vi "set_PulseWidth_subvi.vi"(8 "error in (no error)":errorcluster, 9 "Pulsewidth":dbl, 10 "Aardvark Handle":i32 min=0, 11 "Address (0x50) in":u16=80 max=1023 format="%.0x") -> (0 "error out":errorcluster)   [LabVIEW 2014]
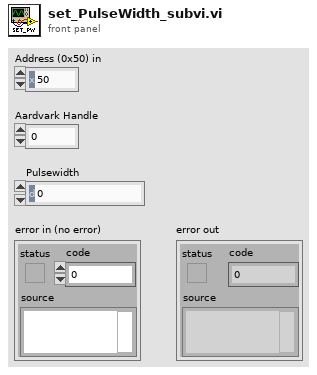
[diagram p1: front panel]
types:
  T1 = cluster{"unsigned byte array[0]":u8, "unsigned byte array[1]":u8, "unsigned byte array[2]":u8, "unsigned byte array[3]":u8, "unsigned byte array[4]":u8, "unsigned byte array[5]":u8, "unsigned byte array[6]":u8, "unsigned byte array[7]":u8, "unsigned byte array[8]":u8}
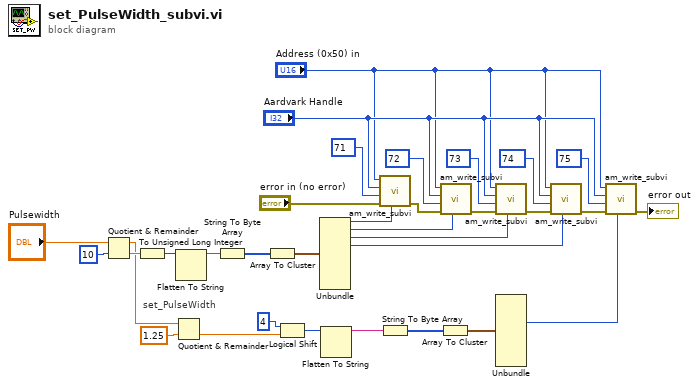
[diagram p0: block diagram]
diagram:
  # "set_PulseWidth"
  n1 = Quotient & Remainder(x="Pulsewidth", y=10) -> (x-y*floor(x/y)=w3:dbl, floor(x/y)=w10:dbl)
  n2 = To Unsigned Long Integer(number=w10) -> (unsigned 32bit integer=w11:u32)
  n3 = Quotient & Remainder(x=w3, y=1.25) -> (floor(x/y)=w6:dbl)  [unwired: 1 out]
  n4 = Flatten To String(anything=w11) -> (data string=w7:string)  [unwired: 3 in, 2 out]
  n5 = String To Byte Array(string=w7) -> (unsigned byte array=w12:u8[])
  n6 = Array To Cluster(array=w12) -> (cluster=w13:T1)
  n7 = Logical Shift(y=4, x=w6) -> (x << y=w9:u32)
  n8 = Unbundle(w13) -> ("unsigned byte array[0]"=w29:u8, "unsigned byte array[1]"=w30:u8, "unsigned byte array[2]"=w31:u8, "unsigned byte array[3]"=w32:u8)  [unwired: 5 out]
  n9 = Flatten To String(anything=w9) -> (data string=w8:string)  [unwired: 3 in, 2 out]
  n10 = call "am_write_subvi.vi"("Data to Write"=w29, "error in (no error)"="error in (no error)", "Memory ADD"=u16 71, "Aardvark Handle in"="Aardvark Handle", "Address (0x50) in"="Address (0x50) in") -> ("error out"=w17:errorcluster)  [unwired: 5 in, 1 out]
  n11 = String To Byte Array(string=w8) -> (unsigned byte array=w14:u8[])
  n12 = Array To Cluster(array=w14) -> (cluster=w15:T1)
  n13 = call "am_write_subvi.vi"("Data to Write"=w30, "error in (no error)"=w17, "Memory ADD"=u16 72, "Aardvark Handle in"="Aardvark Handle", "Address (0x50) in"="Address (0x50) in") -> ("error out"=w18:errorcluster)  [unwired: 5 in, 1 out]
  n14 = call "am_write_subvi.vi"("Data to Write"=w31, "error in (no error)"=w18, "Memory ADD"=u16 73, "Aardvark Handle in"="Aardvark Handle", "Address (0x50) in"="Address (0x50) in") -> ("error out"=w19:errorcluster)  [unwired: 5 in, 1 out]
  n15 = Unbundle(w15) -> ("unsigned byte array[3]"=w33:u8)  [unwired: 8 out]
  n16 = call "am_write_subvi.vi"("Data to Write"=w32, "error in (no error)"=w19, "Memory ADD"=u16 74, "Aardvark Handle in"="Aardvark Handle", "Address (0x50) in"="Address (0x50) in") -> ("error out"=w20:errorcluster)  [unwired: 5 in, 1 out]
  n17 = call "am_write_subvi.vi"("Data to Write"=w33, "error in (no error)"=w20, "Memory ADD"=u16 75, "Aardvark Handle in"="Aardvark Handle", "Address (0x50) in"="Address (0x50) in") -> ("error out"=→"error out":errorcluster)  [unwired: 5 in, 1 out]
